vi "Abort Sub3.vi"(11 "Test Case In":refnum<class "Tests Event MessengerM.lvclass">) -> (0 "error out":errorcluster, 3 "Test Case Out":refnum<class "Tests Event MessengerM.lvclass">)   [LabVIEW 2020, in "Tests Event MessengerM.lvclass"]
uses:
  Tests Event MessengerM.lvclass
  Tests Event MessengerM.lvclass/Tests Event MessengerM.ctl
  C:/Program Files/National Instruments/LabVIEW 2026/vi.lib/Astemes/LUnit/Test Case.lvclass
  C:/Program Files/National Instruments/LabVIEW 2026/vi.lib/Astemes/LUnit/LUnit Runnable.lvclass
  D:/git/Event-MessengerM-Channel-Wire/tests/Tests Event MessengerM/Tests Event MessengerM.lvclass
  <vilib>/Astemes/LUnit/Test Case.lvclass
  52dcce1f-d5b3-4bba-b047-85543a60d1da.vi
  6efbecfc-24dc-4bc3-8dd6-1ca9a130957a.vi
  84629ccf-a762-41c1-860c-8fc252825217.vi
  21970b32-d37a-48e3-a7f3-4205c57ddbaa.vi
  ed77fd87-7123-4487-ad96-f98cf2f41135.vi
  e81c197b-a757-43ac-a7e9-bc63f34c52b5.vi
  af330354-6ddd-49a8-a3f4-3a5d7e93a35e.vi
panel:
  out "cmd 3":string
  out "cmd 2":string
  out "cmd":string
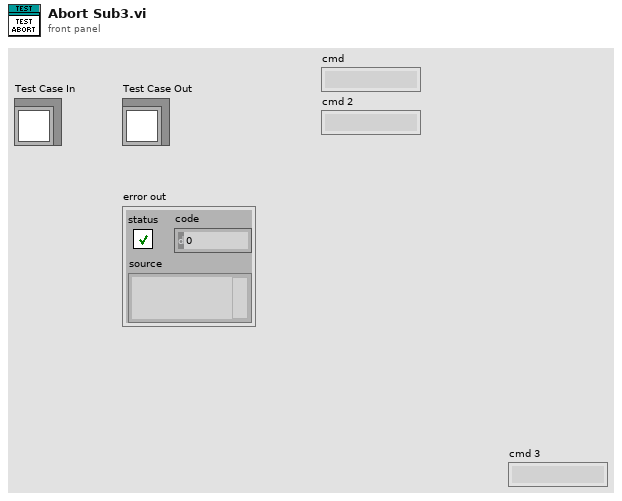
[diagram p1: front panel]
types:
  T1 = typedef "Event MessengerM-c(str,var).lvlib/))Channel.ctl" = refnum<queue>
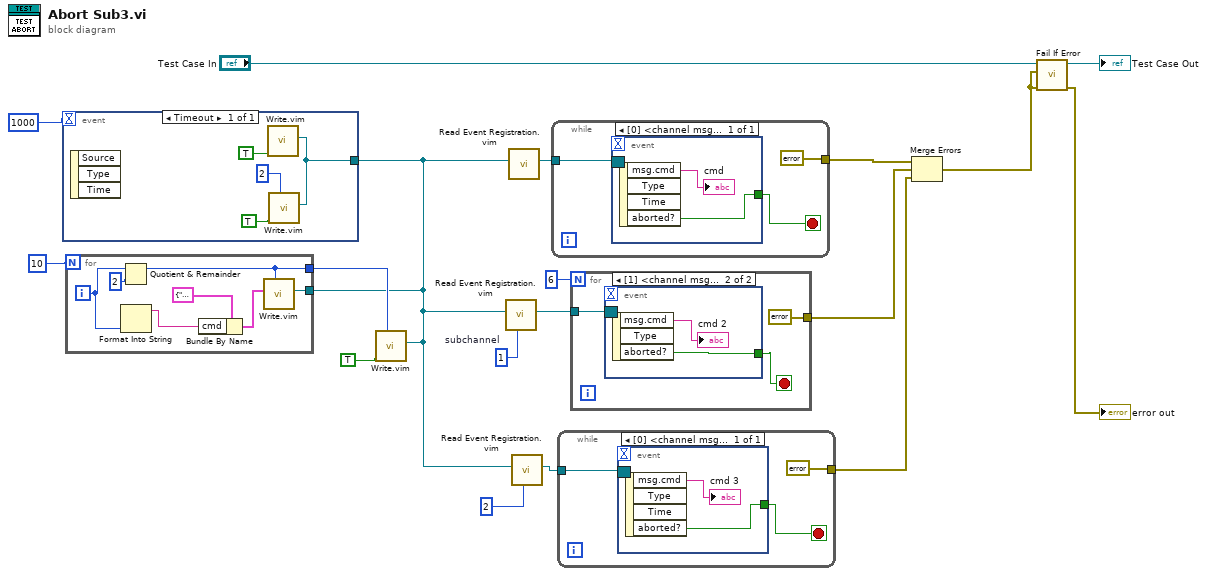
[diagram p0: block diagram]
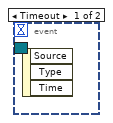
[diagram p2: hidden frame]
diagram:
  w1 = 1  # subchannel
  n1 = for {
    N: 10 -> [_]
    tunnel: [w19] -> w8
    tunnel: [w20] -> w3
    i -> [w23]
    n2 = Quotient & Remainder(x=w23, y=2) -> (x-y*floor(x/y)=w19:i32)  [unwired: 1 out]
    n3 = Format Into String(w23) -> (resulting string=w22:string)  [unwired: 3 in, 1 out]
    n4 = Bundle By Name(cluster=cluster{"cmd":string, "data":variant} {"cmd"="", "data"=variant} ("element"), "cmd"=w22) -> (w21:cluster{"cmd":string, "data":variant})
    n5 = call "Write.vim"("subchannel"=w19, "element"=w21) -> ("channel"=w20:T1)  [unwired: 8 in, 1 out]
  }
  n6 = event shown="[0] Timeout" {
    selector: _ -> [_]
    dyn-events: _ -> [_]
    timeout: 1000 -> [_]
    tunnel: w3 -> [w28]
    event Timeout {
      n7 = event-data() -> ()  [unwired: 1 in, 3 out]
      n8 = call "Write.vim"("abort sub (F)"=TRUE) -> ("channel"=w28:T1)  [unwired: 9 in, 1 out]
      n9 = call "Write.vim"("channel"=w28, "subchannel"=2 ("subchannel (0)"), "abort sub (F)"=TRUE) -> ()  [unwired: 8 in, 1 out]
    }
  }
  n10 = call "Write.vim"("channel"=w3, "subchannel"=w8, "abort sub (F)"=TRUE) -> ()  [unwired: 8 in, 1 out]
  n11 = call "Read Event Registration.vim"("subchannel"=w1, "channel"=w3) -> ("event registration refnum"=w7:refnum<event-registration>)  [unwired: 9 in]
  n12 = call "Read Event Registration.vim"("channel"=w3) -> ("event registration refnum"=w6:refnum<event-registration>)  [unwired: 10 in]
  n13 = call "Read Event Registration.vim"("subchannel"=2 ("subchannel (0)"), "channel"=w3) -> ("event registration refnum"=w4:refnum<event-registration>)  [unwired: 9 in]
  n14 = while {
    tunnel: w6 -> [w32]
    tunnel: [errorcluster {"status"=FALSE, "code"=0, "source"=""} ("error constant")] -> w12
    stop <- w31 stop-if-true
    n15 = event shown="[0] <channel msg>: User Event" {
      selector: w32 -> [_]
      dyn-events: _ -> [_]
      timeout: _ -> [_]
      tunnel: [w33] -> w31
      event User Event {
        n16 = event-data() -> ("msg.cmd"=→"cmd":string, "aborted?"=w33:bool)  [unwired: 1 in, 2 out]
      }
    }
  }
  n17 = while {
    tunnel: w4 -> [w37]
    tunnel: [errorcluster {"status"=FALSE, "code"=0, "source"=""} ("error constant")] -> w5
    stop <- w36 stop-if-true
    n18 = event shown="[0] <channel msg>: User Event" {
      selector: w37 -> [_]
      dyn-events: _ -> [_]
      timeout: _ -> [_]
      tunnel: [w38] -> w36
      event User Event {
        n19 = event-data() -> ("msg.cmd"=→"cmd 3":string, "aborted?"=w38:bool)  [unwired: 1 in, 2 out]
      }
    }
  }
  n20 = for {
    N: 6 -> [_]
    tunnel: w7 -> [w42]
    tunnel: [errorcluster {"status"=FALSE, "code"=0, "source"=""} ("error constant")] -> w11
    stop <- w41 stop-if-true
    n21 = event shown="[1] <channel msg>: User Event" {
      selector: w42 -> [_ _]
      dyn-events: _ -> [_ _]
      timeout: _ -> [_ _]
      tunnel: [_ w43] -> w41
      event Timeout {
        n22 = event-data() -> ()  [unwired: 1 in, 3 out]
      }
      event User Event {
        n23 = event-data() -> ("msg.cmd"=→"cmd 2":string, "aborted?"=w43:bool)  [unwired: 1 in, 1 out]
      }
    }
  }
  n24 = Merge Errors(w12, w11, w5) -> (w10:errorcluster)
  n25 = call <vilib>:"Fail If Error.vi"("error in (no error)"=w10, "Assert error"=w10, "LUnit Test Case In"="Test Case In") -> ("error out"=→"error out":errorcluster, "LUnit Test Case Out"=→"Test Case Out":refnum<class "Tests Event MessengerM.lvclass">)  [unwired: 7 in]
